vi "波形图.vi"() -> ()   [LabVIEW 2018]
panel:
  out "波形图 3":cluster{dbl, dbl, dbl[]}(graph)
  out "波形图 2":dbl[][](graph)
  out "波形图":dbl[](graph)
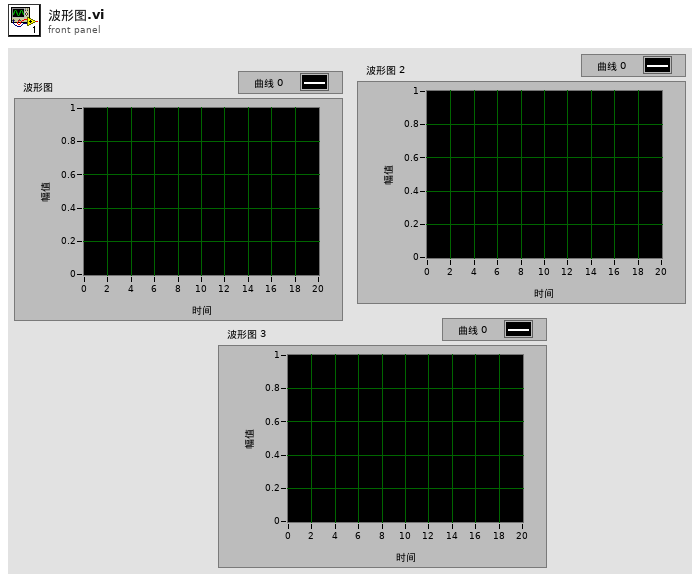
[diagram p1: front panel]
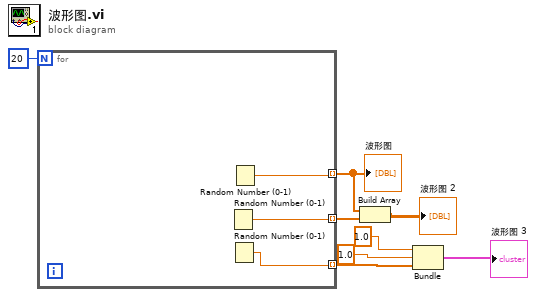
[diagram p0: block diagram]
diagram:
  n1 = for {
    N: 20 -> [_]
    tunnel: [w11] -> w5 mode=indexing
    tunnel: [w10] -> w7 mode=indexing
    tunnel: [w9] -> w4 mode=indexing
    n2 = Random Number (0-1)() -> (number: 0 to 1=w10:dbl)
    n3 = Random Number (0-1)() -> (number: 0 to 1=w9:dbl)
    n4 = Random Number (0-1)() -> (number: 0 to 1=w11:dbl)
  }
  "波形图" <- w5
  n5 = Build Array(w5, w7) -> (→"波形图 2":dbl[][])
  n6 = Bundle(1.0, 1.0, w4) -> (→"波形图 3":cluster{dbl, dbl, dbl[]})  [unwired: 1 in]
